vi "initializeRun.vi"(7 "xwpfRun in":refnum<class "xwpfRun.lvclass">=refnum, 8 "error in (no error)":errorcluster, 11 "Run Ref":refnum<k24>) -> (0 "error out":errorcluster, 3 "xwpfRun out":refnum<class "xwpfRun.lvclass">)   [LabVIEW 2017]
uses:
  xwpfRun.lvclass
  C:/Users/Neo/Desktop/Dev_Tools_BR/LabVIEW_NPOI/lib/NPOI 2.1.1/NPOI.OOXML.dll
  lib/NPOI 2.1.1/NPOI.OOXML.dll
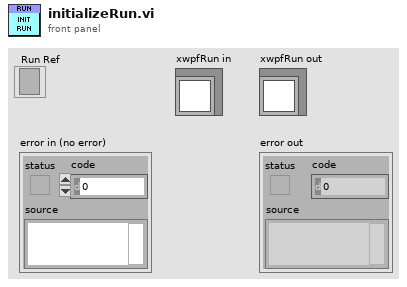
[diagram p1: front panel]
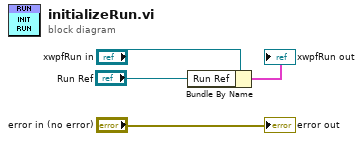
[diagram p0: block diagram]
diagram:
  n1 = Bundle By Name(cluster="xwpfRun in", "Run Ref"="Run Ref") -> (→"xwpfRun out":cluster{})
  "error out" <- "error in (no error)"
